vi "Zustand aendern.vi"(10 "Zustand":T1) -> (2 "Zustand":T1)   [LabVIEW 2020, in "Funktionstasten.lvlib"]
uses:
  Funktionstasten.lvlib
  Zustaende.ctl
  Funktionstasten-Aktion.ctl
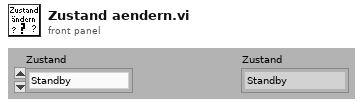
[diagram p1: front panel]
types:
  T1 = typedef "Funktionstasten.lvlib/Zustaende.ctl" = enum16{"Standby", "Pause", "Eco", "Messen", "Kalibrieren", "Spülen Filter", "Spülen Leitung", "Umgebungsluft", "0-Gas", "Cal-Gas", "CG zu PNS", "-------------", "Init 1", "Init 2", "Init 3", "Init 4", "Messen vorbereiten", "Messen durchführen", "Exit"}
  T2 = typedef "Funktionstasten.lvlib/Funktionstasten-Aktion.ctl" = enum16{"Initialisieren", "Zustand setzen", "Taste gedrückt", "Fehler speichern", "Lesen", "Manuell", "Remote", "Bitparallel", "Samplepoint", "Zeit Prüfen", "reset Umschalten"}
  T3 = typedef "Funktionstasten.lvlib/Betriebsart.ctl" = enum16{"Manuell", "Remote", "Bitparallel"}
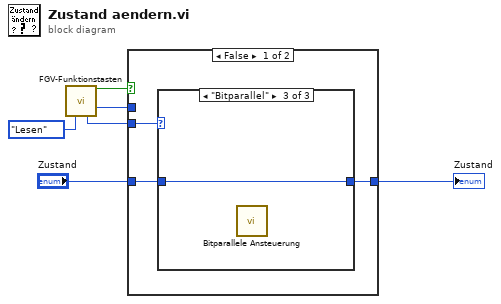
[diagram p0: block diagram]
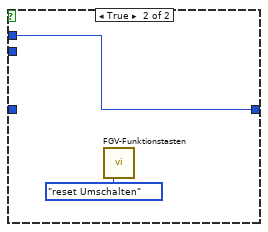
[diagram p4: hidden frame]
diagram:
  n1 = call "FGV-Funktionstasten.vi"("Aktion"=Funktionstasten-Aktion."Lesen") -> ("EXTERN Umschalten"=w5:bool, "ausgewählte Funktion"=w3:T1, "Betriebsart"=w1:T3)  [unwired: 7 in, 5 out]
  n2 = case shown="False" w5 {
    tunnel: "Zustand" -> [w9 _]
    tunnel: [w7 w13] -> w2
    tunnel: w3 -> [_ w13]
    tunnel: w1 -> [w8 _]
    frame False {
      n3 = case shown="\"Bitparallel\"" w8 {
        tunnel: w9 -> [w10 w11 w12]
        tunnel: [w10 w11 w12] -> w7
        frame "Manuell", Default {
        }
        frame "Remote" {
        }
        frame "Bitparallel" {
          n4 = call "Bitparallele Ansteuerung.vi"() -> ()  [unwired: 12 in]
        }
      }
    }
    frame True {
      n5 = call "FGV-Funktionstasten.vi"("Aktion"=Funktionstasten-Aktion."reset Umschalten") -> ()  [unwired: 7 in, 8 out]
    }
  }
  "Zustand" <- w2
